vi "Tables.vi"(8 "1D Array":u64[](array[numeric]), 10 "Numeric":i64, 11 "2D Array":u64[][](array[numeric])) -> (0 "1D Table Control":string[][](table), 3 "2D Table Control":string[][](table))   [LabVIEW 2023]
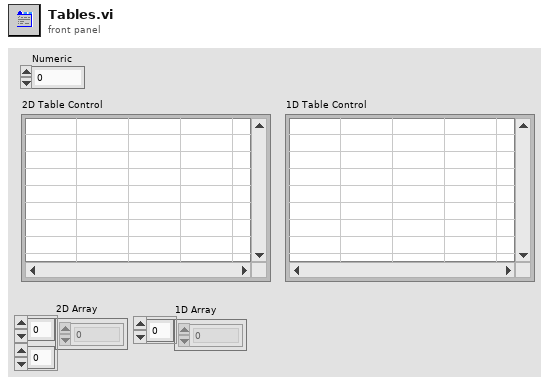
[diagram p1: front panel]
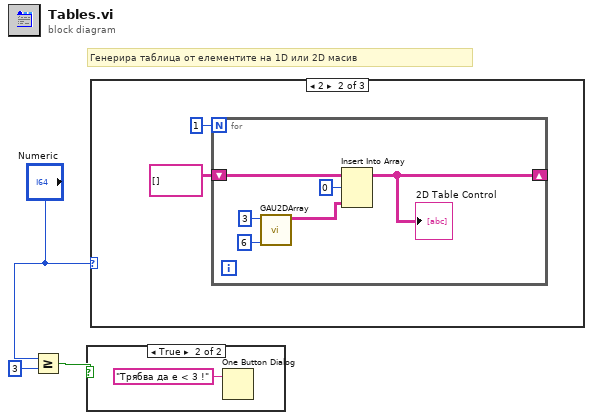
[diagram p0: block diagram]
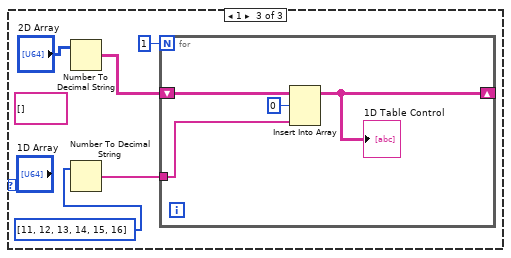
[diagram p4: hidden frame]
diagram:
  # "Генерира таблица от елементите на 1D или 2D масив"
  n1 = Greater Or Equal?(x="Numeric", y=i64 3) -> (x >= y?=w1:bool)
  n2 = case shown="True" w1 {
    frame False {
    }
    frame True {
      n3 = One Button Dialog(message="Трябва да е < 3 !") -> ()  [unwired: 1 in, 1 out]
    }
  }
  n4 = case shown="2" "Numeric" {
    frame 0, Default {
    }
    frame 2 {
      n5 = for {
        N: 1 -> [_]
        shift-right: [w7] -> _
        shift-left: string[][] [] -> [w12]
        n6 = call "GAU2DArray.vi"("Colums"=6, "Rows"=3) -> ("2D String Array"=w8:string[][])  [unwired: 8 in, 1 out]
        n7 = Insert Into Array "Insert Into Array"(array=w12, index (row)=0 ("index"), new element=w8) -> (w7:string[][])  [unwired: 1 in]
        "2D Table Control" <- w7
      }
    }
    frame 1 {
      (unwired) string[][] []
      n8 = Number To Decimal String(number="2D Array") -> (decimal integer string=w15:string[][])  [unwired: 1 in]
      n9 = Number To Decimal String(number=i32[] [11, 12, 13, 14, 15, 16]) -> (decimal integer string=w14:string[])  [unwired: 1 in]
      n10 = for {
        N: 1 -> [_]
        shift-right: [w19] -> _
        shift-left: w15 -> [w21]
        tunnel: w14 -> [w18]
        n11 = Insert Into Array "Insert Into Array"(array=w21, index (row)=0 ("index"), new element=w18) -> (w19:string[][])  [unwired: 1 in]
        "1D Table Control" <- w19
      }
    }
  }
